vi "Temperature Monitor.vi"() -> ()   [LabVIEW 2017]
doc: "This VI is the solution to an exercise in the LabVIEW Core 1 course.\n\nIt uses a While Loop and shift registers to average data. No hardware is necessary."
panel:
  in  "Stop Button":bool
  out "Temperature History":cluster{dbl, "Temperature Value":dbl}(graph)
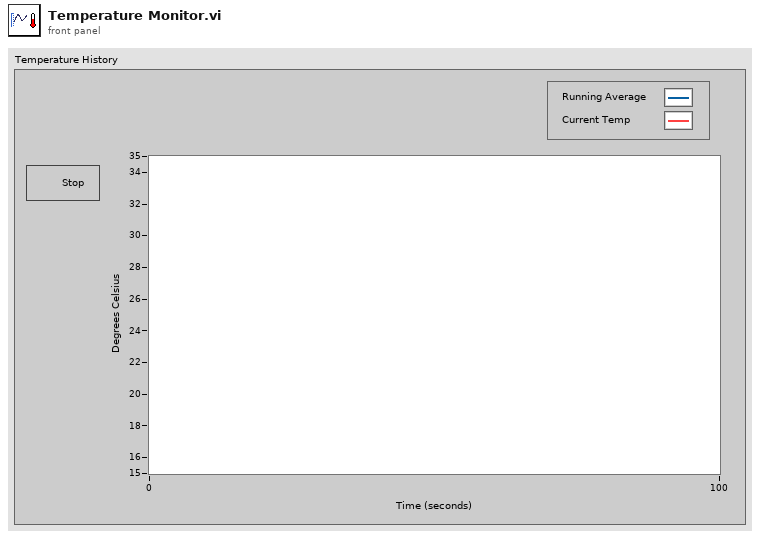
[diagram p1: front panel]
types:
  T1 = enum16{"open", "replace", "create", "open or create", "replace or create", "replace or create with confirmation"}
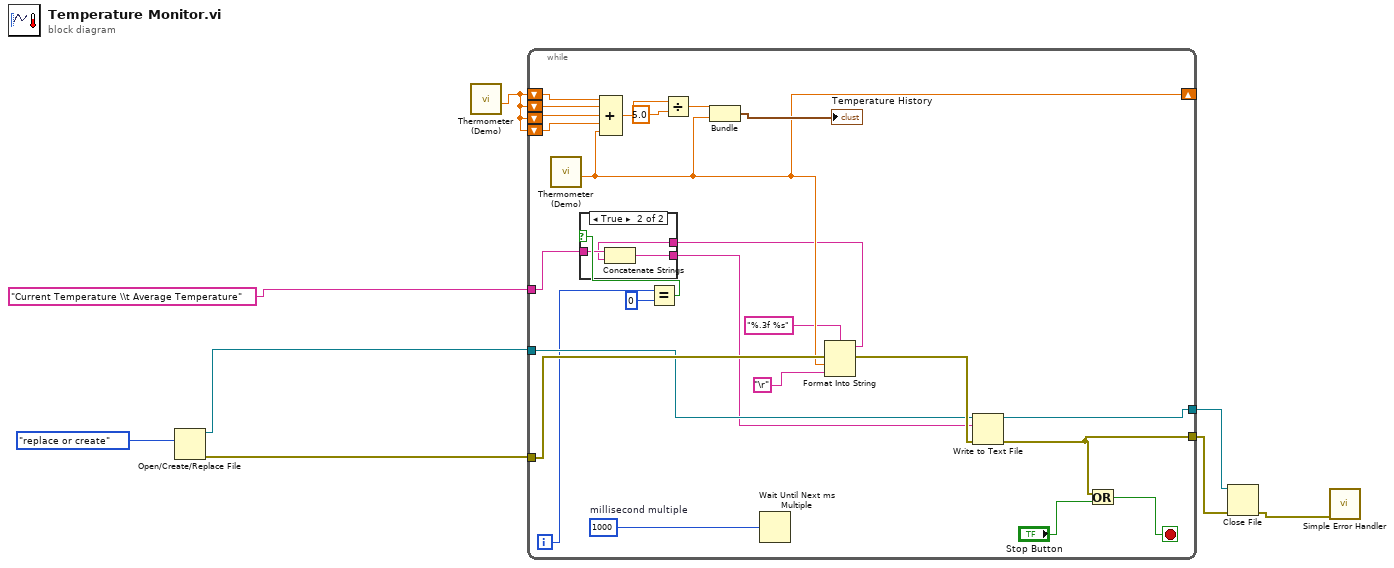
[diagram p0: block diagram]
diagram:
  n1 = Open/Create/Replace File(operation (0:open)=T1."replace or create") -> (refnum out=w7:refnum<file>, error out=w1:errorcluster)  [unwired: 5 in, 1 out]
  n2 = call "Thermometer (Demo).vi"() -> ("Temperature Value"=w8:dbl)  [unwired: 11 in]
  n3 = while {
    shift-right: [w22] -> _
    shift-left: w8 -> [w32]
    shift-left: w8 -> [w31]
    shift-left: w8 -> [w30]
    shift-left: w8 -> [w29]
    tunnel: w1 -> [w24]
    tunnel: w7 -> [w16]
    tunnel: [w18] -> w5
    tunnel: [w17] -> w4
    tunnel: "Current Temperature \\t Average Temperature" ("text") -> [w14]
    i -> [w13]
    stop <- w20 stop-if-true
    w33 = u32 1000  # millisecond multiple
    n4 = call "Thermometer (Demo).vi"() -> ("Temperature Value"=w22:dbl)  [unwired: 11 in]
    n5 = Compound Arithmetic op=ADD(w32, w31, w30, w29, w22) -> (w28:dbl)
    n6 = Equal?(x=w13, y=0) -> (x = y?=w11:bool)
    n7 = Divide(x=w28, y=5.0) -> (x/y=w26:dbl)
    n8 = Bundle(w26, "Temperature Value"=w22) -> (→"Temperature History":cluster{dbl, "Temperature Value":dbl})  [unwired: 1 in]
    n9 = Wait Until Next ms Multiple(millisecond multiple=w33) -> ()  [unwired: 1 out]
    n10 = Format Into String "Format Into String"(format string="%.3f %s", error in=w24, w22, "\r") -> (resulting string=w10:string, error out=w21:errorcluster)  [unwired: 1 in]
    n11 = case shown="True" w11 {
      tunnel: w14 -> [_ w37]
      tunnel: w10 -> [w34 w36]
      tunnel: [w34 w35] -> w9
      frame False {
      }
      frame True {
        n12 = Concatenate Strings(w37, w36) -> (w35:string)
      }
    }
    n13 = Write to Text File(file (use dialog)=w16, text=w9, error in=w21) -> (refnum out=w17:refnum<file>, error out=w18:errorcluster)  [unwired: 1 in, 1 out]
    n14 = Or(x=w18, y="Stop Button") -> (x .or. y?=w20:bool)
  }
  n15 = Close File(refnum=w4, error in=w5) -> (error out=w3:errorcluster)  [unwired: 1 out]
  n16 = call <vilib>:"Simple Error Handler.vi"("error in (no error)"=w3) -> ()  [unwired: 4 in, 5 out]
